vi "prepare_position_overlay.vi"(8 "error in (no error)":errorcluster, 10 "position channels":T1, 11 "Image in":refnum<class "Image.lvclass">) -> (0 "error out":errorcluster, 2 "pixel positions":T2, 3 "Image out":refnum<class "Image.lvclass">)   [LabVIEW 2010, in "Image.lvclass"]
uses:
  Image.lvclass
  pixel_positions_cluster.ctl
  position_channels_cluster.ctl
  Image.lvclass/Image.ctl
  ErrorController/ErrorController/class_data.vi
  <vilib>/Analysis/NI_AALBase.lvlib
  ErrorController/ErrorController/ErrorController.lvclass
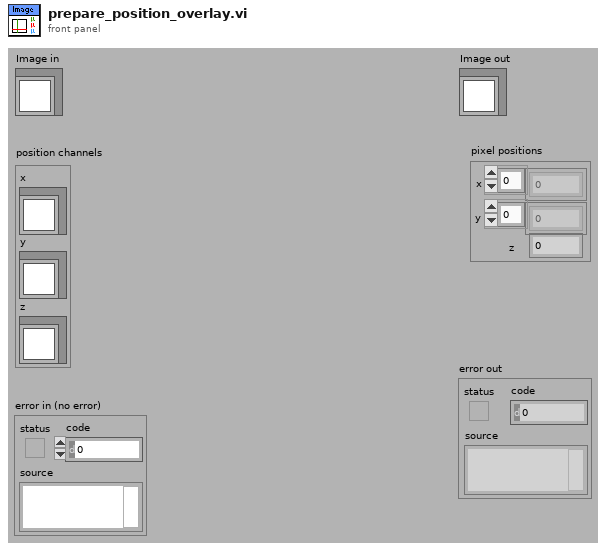
[diagram p1: front panel]
types:
  T1 = typedef "Image.lvclass/position_channels_cluster.ctl" = cluster{"x":refnum<class "Image.lvclass">, "y":refnum<class "Image.lvclass">, "z":refnum<class "Image.lvclass">}
  T2 = typedef "Image.lvclass/pixel_positions_cluster.ctl" = cluster{"x":dbl[], "y":dbl[], "z":dbl}
  T3 = typedef "IMAQ Image.ctl" = refnum<image>
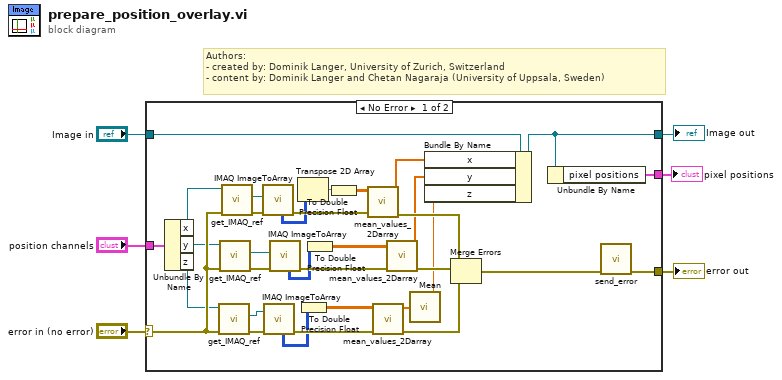
[diagram p0: block diagram]
diagram:
  # "Authors: \n- created by: Dominik Langer, University of Zurich, Switzerland\n- content by: Dominik Langer and Chetan Nagaraja (University of Uppsala, Sweden)"
  n1 = case shown="No Error" "error in (no error)" {
    selector: "error in (no error)" -> [w23 w41]
    tunnel: [w7 w41] -> w5
    tunnel: [w14 w40] -> w3
    tunnel: "Image in" -> [w18 w40]
    tunnel: [w13 _] -> w2
    tunnel: "position channels" -> [w12 _]
    frame No Error {
      n2 = Unbundle By Name(w12) -> ("x"=w9:refnum<class "Image.lvclass">, "y"=w10:refnum<class "Image.lvclass">, "z"=w11:refnum<class "Image.lvclass">)
      n3 = call-dynamic "get_IMAQ_ref.vi"("error in (no error)"=w23, "Image.lvclass in"=w11) -> ("error out"=w39:errorcluster, "Image"=w35:T3)  [unwired: 5 in, 3 out]
      n4 = call-dynamic "get_IMAQ_ref.vi"("error in (no error)"=w23, "Image.lvclass in"=w10) -> ("error out"=w33:errorcluster, "Image"=w30:T3)  [unwired: 5 in, 3 out]
      n5 = call-dynamic "get_IMAQ_ref.vi"("error in (no error)"=w23, "Image.lvclass in"=w9) -> ("error out"=w29:errorcluster, "Image"=w25:T3)  [unwired: 5 in, 3 out]
      n6 = call "IMAQ ImageToArray"("error in (no error)"=w29, "Image"=w25) -> ("Image Pixels (U16)"=w24:u16[][], "error out"=w28:errorcluster)  [unwired: 2 in, 3 out]
      n7 = call "IMAQ ImageToArray"("error in (no error)"=w39, "Image"=w35) -> ("Image Pixels (U16)"=w34:u16[][], "error out"=w38:errorcluster)  [unwired: 2 in, 3 out]
      n8 = call "IMAQ ImageToArray"("error in (no error)"=w33, "Image"=w30) -> ("Image Pixels (U16)"=w22:u16[][], "error out"=w32:errorcluster)  [unwired: 2 in, 3 out]
      n9 = Transpose 2D Array(2D array=w24) -> (transposed array=w27:u16[][])
      n10 = To Double Precision Float(number=w34) -> (double precision float=w37:dbl[][])
      n11 = To Double Precision Float(number=w22) -> (double precision float=w31:dbl[][])
      n12 = To Double Precision Float(number=w27) -> (double precision float=w26:dbl[][])
      n13 = call "mean_values_2Darray.vi"("error in (no error)"=w28, "Array"=w26) -> ("error out"=w21:errorcluster, "mean values"=w17:dbl[])  [unwired: 6 in]
      n14 = call "mean_values_2Darray.vi"("error in (no error)"=w38, "Array"=w37) -> ("error out"=w19:errorcluster, "mean values"=w36:dbl[])  [unwired: 6 in]
      n15 = call "mean_values_2Darray.vi"("error in (no error)"=w32, "Array"=w31) -> ("error out"=w20:errorcluster, "mean values"=w16:dbl[])  [unwired: 6 in]
      n16 = call <vilib>:"Mean.vi"("X"=w36) -> ("mean"=w15:dbl)  [unwired: 1 out]
      n17 = Bundle By Name(cluster=w18, "x"=w17, "y"=w16, "z"=w15) -> (w14:refnum<class "Image.lvclass">)
      n18 = Merge Errors(w21, w20, w19) -> (w8:errorcluster)
      n19 = Unbundle By Name(w14) -> ("pixel positions"=w13:T2)
      n20 = call "send_error.vi"("error in (no error)"=w8) -> ("error out"=w7:errorcluster)  [unwired: 10 in]
    }
    frame Error {
    }
  }
  "error out" <- w5
  "Image out" <- w3
  "pixel positions" <- w2
